vi "Main.vi"   [LabVIEW 2017]
doc: "The start-up VI for our application and the UI"
types:
  T1 = typedef "View Model.ctl" = cluster{"Error Model":T2, "Shared Model":T3, "Elevator Model":T4, "Configuration Model":T5}
  T2 = typedef "Error Model.ctl" = cluster{"Error Event":refnum<user-event>}
  T3 = typedef "Shared Model.ctl" = cluster{"Stop DVR":refnum<data-value>, "Stop Event":refnum<user-event>}
  T4 = typedef "Elevator Model.ctl" = cluster{"Controller Overhead":refnum<data-value>, "Motion Change":refnum<user-event>, "Direction Change":refnum<user-event>, "Door Position Change":refnum<user-event>, "Emergency Change":refnum<user-event>, "Floor Change":refnum<user-event>, "Elevator Cmd":refnum<user-event>}
  T5 = typedef "Configuration Model.ctl" = cluster{"Configuration":refnum<data-value>, "Config Change":refnum<user-event>}
  T6 = enum32{"invalid app kind", "Development System", "Run Time System", "Student Edition", "Embedded LabVIEW", "Evaluation", "Custom"}
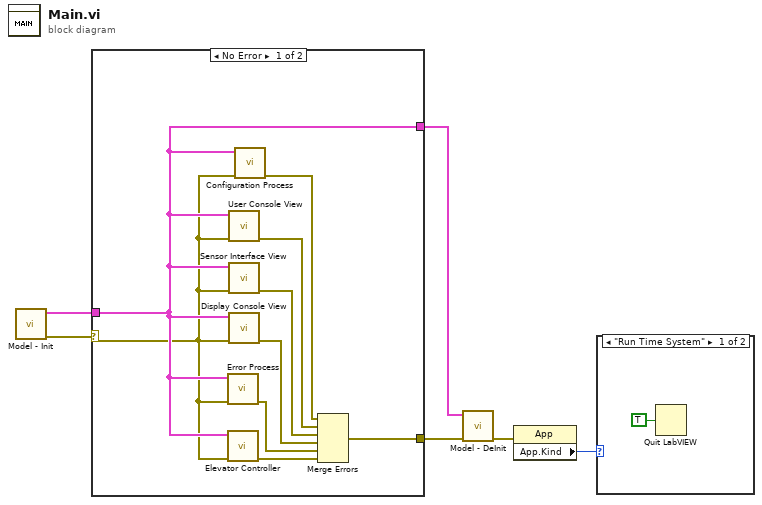
[diagram p0: block diagram]
diagram:
  n1 = call "Model - Init.vi"() -> ("error out"=w5:errorcluster, "View Model"=w6:T1)  [unwired: 10 in]
  n2 = case shown="No Error" w5 {
    selector: w5 -> [w8 w16]
    tunnel: w6 -> [w9 w17]
    tunnel: [w10 w16] -> w3
    tunnel: [w9 w17] -> w1
    frame No Error {
      n3 = call "Error Process.vi"("error in (no error)"=w8, "View Model"=w9) -> ("error out"=w14:errorcluster)  [unwired: 9 in]
      n4 = call "Elevator Controller.vi"("error in (no error)"=w8, "View Model"=w9) -> ("error out"=w15:errorcluster)  [unwired: 9 in]
      n5 = call "User Console View.vi"("error in (no error)"=w8, "View Model"=w9) -> ("error out"=w11:errorcluster)  [unwired: 9 in]
      n6 = call "Sensor Interface View.vi"("error in (no error)"=w8, "View Model"=w9) -> ("error out"=w12:errorcluster)  [unwired: 8 in, 1 out]
      n7 = call "Display Console View.vi"("error in (no error)"=w8, "View Model"=w9) -> ("error out"=w13:errorcluster)  [unwired: 9 in]
      n8 = call "Configuration Process.vi"("error in (no error)"=w8, "View Model"=w9) -> ("error out"=w7:errorcluster)  [unwired: 9 in]
      n9 = Merge Errors(w7, w11, w12, w13, w14, w15) -> (w10:errorcluster)
    }
    frame Error {
    }
  }
  n10 = call "Model - DeInit.vi"("error in (no error)"=w3, "View Model"=w1) -> ("error out"=w2:errorcluster)  [unwired: 9 in]
  n11 = property class="App"(error in=w2) -> ("App.Kind"=w4:T6)  [unwired: 1 in, 2 out]
  n12 = case shown="\"Run Time System\"" w4 {
    frame "Run Time System" {
      n13 = Quit LabVIEW(quit? (T)=TRUE) -> ()
    }
    frame "Development System", Default {
    }
  }
